vi "Initialize AI Task.vi"(8 "error in (no error)":errorcluster, 11 "BNT_DAQmx-MCSV-I in":refnum<class "BNT_DAQmx-MCSV-I.lvclass">) -> (0 "error out":errorcluster, 3 "AI DAQmx Task":refnum<k21>)   [LabVIEW 2020, in "BNT_DAQmx.lvlib" / "BNT_DAQmx-MCSV-I.lvclass"]
doc: "Initialize DAQmx Analog Input task. Every derived class needs to start the task on its own.\n\n<b>Default Implementation:</b> Analog Input Current\n\nThis dynamic dispatch VI can be overritten by derived classes to implement other analog input tasks."
uses:
  BNT_DAQmx-MCSV-I.lvclass
  BNT_DAQmx-MCSV-I.lvclass/BNT_DAQmx-MCSV-I.ctl
  <vilib>/DAQmx/create/channels.llb/DAQmx Create Channel (AI-Current-Basic).vi
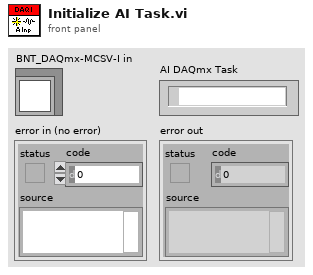
[diagram p1: front panel]
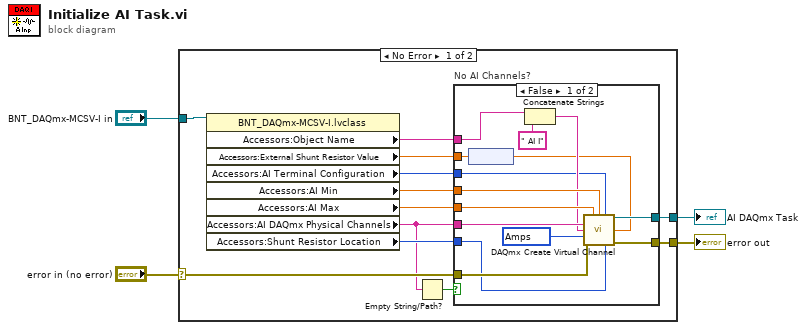
[diagram p0: block diagram]
diagram:
  n1 = case shown="No Error" "error in (no error)" {
    selector: "error in (no error)" -> [w16 w32]
    tunnel: [w8 w32] -> w1
    tunnel: "BNT_DAQmx-MCSV-I in" -> [w15 _]
    tunnel: [w9 _] -> w2
    frame No Error {
      n2 = property class="BNT_DAQmx-MCSV-I.lvclass"(reference=w15) -> ("Accessors:Object Name"=w7:string, "Accessors:External Shunt Resistor Value"=w11:dbl[unit], "Accessors:AI Terminal Configuration"=w12:i32, "Accessors:AI Min"=w13:dbl, "Accessors:AI Max"=w14:dbl, "Accessors:AI DAQmx Physical Channels"=w6:tag, "Accessors:Shunt Resistor Location"=w10:i32)  [unwired: 1 in, 2 out]
      n3 = Empty String/Path?(string/path=w6) -> (empty?=w5:bool)
      n4 = case "No AI Channels?" shown="False" w5 {
        tunnel: w16 -> [w30 w31]
        tunnel: w6 -> [w29 _]
        tunnel: w14 -> [w28 _]
        tunnel: w13 -> [w27 _]
        tunnel: w12 -> [w19 _]
        tunnel: w11 -> [w18 _]
        tunnel: w10 -> [w26 _]
        tunnel: [w25 _] -> w9
        tunnel: [w24 w31] -> w8
        tunnel: w7 -> [w22 _]
        frame False {
          w20 = 10342 items=["Amps"=10342, "From Custom Scale"=10065] ("units")
          n5 = node(w18) -> (w17:dbl)
          n6 = Concatenate Strings(w22, " AI I" ("string")) -> (w21:string)
          n7 = call-poly <vilib>:"DAQmx Create Virtual Channel.vi"("maximum value"=w28, "minimum value"=w27, "input terminal configuration"=w19, "physical channels"=w29, "name to assign"=w21, "external shunt resistor value"=w17, "units"=w20, "error in"=w30, "shunt resistor location"=w26) -> ("task out"=w25:refnum<k21>, "error out"=w24:errorcluster)  [unwired: 5 in]
        }
        frame True {
        }
      }
    }
    frame Error {
    }
  }
  "error out" <- w1
  "AI DAQmx Task" <- w2
